vi "Parse New Members.vi"(8 "error in (no error)":errorcluster, 10 "Club Members JSON":string, 11 "Data Manager in":refnum<class "Data Manager.lvclass">) -> (0 "error out":errorcluster, 3 "Data Manager out":refnum<class "Data Manager.lvclass">)   [LabVIEW 2020, in "Data Manager.lvclass"]
uses:
  Data Manager.lvclass
  Strava JSON for Club Members--cluster.ctl
  Data Manager.lvclass/Data Manager.ctl
  Name--cluster.ctl
  Profile--cluster.ctl
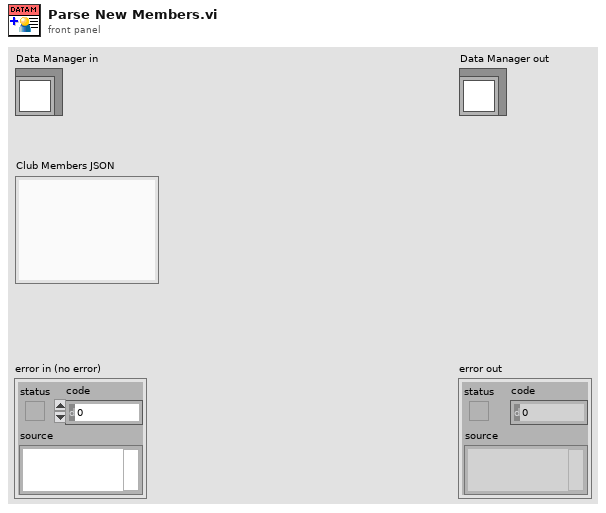
[diagram p1: front panel]
types:
  T1 = typedef "Data Manager.lvclass/Strava JSON for Club Members--cluster.ctl" = cluster{"firstname":string, "lastname":string}
  T2 = typedef "Data Manager.lvclass/Profile--cluster.ctl" = cluster{"Alias":string, "Team":string}
  T3 = typedef "Data Manager.lvclass/Name--cluster.ctl" = cluster{"First":string, "Last":string}
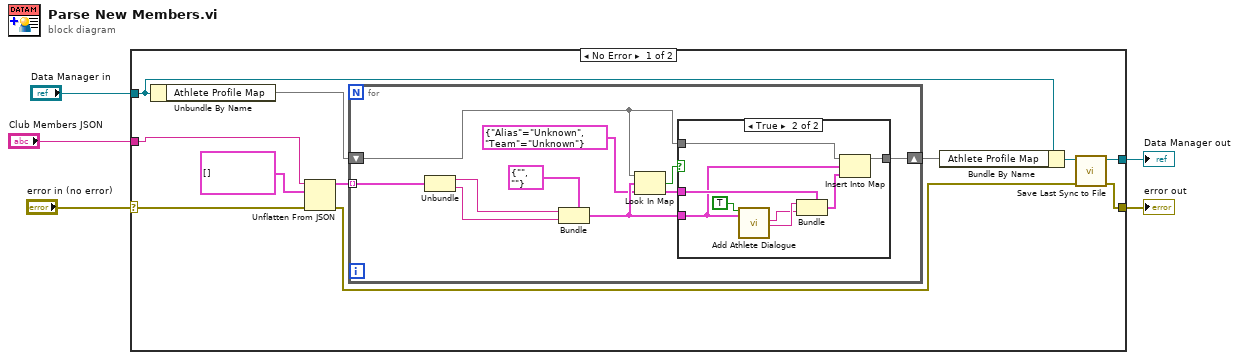
[diagram p0: block diagram]
diagram:
  n1 = case shown="No Error" "error in (no error)" {
    selector: "error in (no error)" -> [w14 w37]
    tunnel: [w12 w37] -> w4
    tunnel: [w13 w36] -> w2
    tunnel: "Data Manager in" -> [w10 w36]
    tunnel: "Club Members JSON" -> [w15 _]
    frame No Error {
      n2 = Unbundle By Name(w10) -> ("Athlete Profile Map"=w8:map{T3, T2})
      n3 = Unflatten From JSON(JSON string=w15, type and defaults=T1[] [], error in (no error)=w14) -> (value=w9:T1[], error out=w6:errorcluster)  [unwired: 4 in]
      n4 = for {
        tunnel: w9 -> [w26] mode=indexing
        shift-right: [w18] -> w7
        shift-left: w8 -> [w19]
        n5 = Unbundle(w26) -> ("firstname"=w21:string, "lastname"=w20:string)
        n6 = Bundle(cluster=T3 {"First"="", "Last"=""} ("Name"), "First"=w21, "Last"=w20) -> (w23:T3)
        n7 = Look In Map(map=w19, key=w23, default value=T2 {"Alias"="Unknown", "Team"="Unknown"}) -> (key not found?=w25:bool, value=w24:T2)
        n8 = case shown="True" w25 {
          tunnel: w19 -> [w27 w35]
          tunnel: [w27 w34] -> w18
          tunnel: w24 -> [_ w33]
          tunnel: w23 -> [_ w31]
          frame False {
          }
          frame True {
            n9 = call "Add Athlete Dialogue.vi"("Enable"=TRUE, "Name"=w31) -> ("Team"=w28:string, "Athlete"=w29:string)  [unwired: 14 in, 2 out]
            n10 = Bundle(cluster=w33, "Alias"=w29, "Team"=w28) -> (w30:T2)
            n11 = Insert Into Map(map in=w35, key=w31, value=w30) -> (map out=w34:map{T3, T2})  [unwired: 2 out]
          }
        }
      }
      n12 = Bundle By Name(cluster=w10, "Athlete Profile Map"=w7) -> (w11:refnum<class "Data Manager.lvclass">)
      n13 = call-dynamic "Save Last Sync to File.vi"("error in (no error)"=w6, "Data Manager in"=w11) -> ("error out"=w12:errorcluster, "Data Manager out"=w13:refnum<class "Data Manager.lvclass">)  [unwired: 8 in]
    }
    frame Error {
    }
  }
  "error out" <- w4
  "Data Manager out" <- w2
